vi "nav3.vi"(9 "Drone":T3, 11 "Field":T1[][](array[typedef])) -> (2 "Move?":bool, 3 "direction":T2 items=["^", "^>", ">", "V>", "V", "<V", "<", "<^"])   [LabVIEW 2009]
uses:
  Drone data.ctl
  direction.ctl
  square.ctl
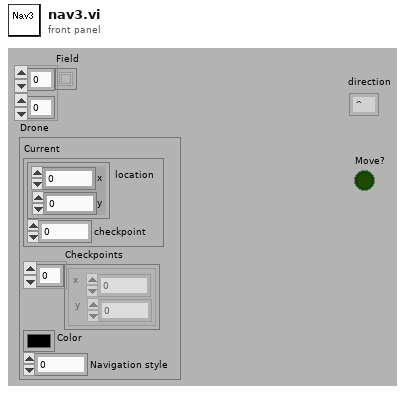
[diagram p1: front panel]
types:
  T1 = typedef "square.ctl" = u8
  T2 = typedef "direction.ctl" = i8
  T3 = typedef "Drone data.ctl" = cluster{"Current":cluster{"location":cluster{"x":i16, "y":i16}, "checkpoint":i32}, "Checkpoints":cluster{"x":i16, "y":i16}[], "Color":u32, "Navigation style":i32}
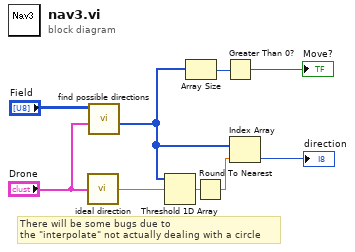
[diagram p0: block diagram]
diagram:
  # "There will be some bugs due to\nthe \"interpolate\" not actually dealing with a circle"
  n1 = call "ideal direction.vi"("Drone"="Drone") -> ("ideal direction"=w7:dbl)
  n2 = call "find possible directions.vi"("Drone"="Drone", "Field"="Field") -> ("possible directions"=w6:T2[])  [unwired: 8 in, 1 out]
  n3 = Threshold 1D Array(2:w7, 3:w6) -> (0:w4:dbl)  [unwired: 1 in]
  n4 = Array Size(array=w6) -> (size(s)=w3:i32)
  n5 = Round To Nearest(number=w4) -> (nearest integer value=w5:dbl)
  n6 = Greater Than 0?(x=w3) -> (x > 0?=→"Move?":bool)
  n7 = Index Array(array=w6, index=w5) -> (element=→"direction":T2)
